vi "ReadBool to ArrayByte.vi"(1 "Items":u16, 2 "Pos":u16) -> (0 "ArrayByte":u16)   [LabVIEW 2014, in "Simatic S7.lvlib"]
uses:
  Simatic S7.lvlib
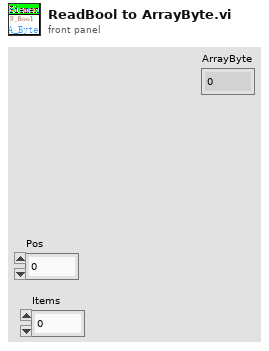
[diagram p1: front panel]
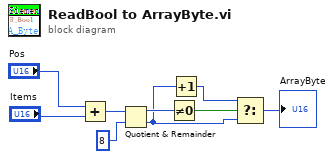
[diagram p0: block diagram]
diagram:
  n1 = Add(x="Pos", y="Items") -> (x+y=w7:u16)
  n2 = Quotient & Remainder(x=w7, y=u16 8) -> (x-y*floor(x/y)=w5:u16, floor(x/y)=w2:u16)
  n3 = Not Equal To 0?(x=w5) -> (x != 0?=w4:bool)
  n4 = Increment(x=w2) -> (x+1=w3:u16)
  n5 = Select(t=w3, s=w4, f=w2) -> (s? t:f=→"ArrayByte":u16)
